vi "Pengukuran WHS 4 Ch.vi"() -> ()   [LabVIEW 2018]
uses:
  <vilib>/Utility/error.llb/DialogType.ctl
  <vilib>/DAQmx/read.llb/DAQmx Read (Analog 1D Wfm NChan NSamp).vi
  <vilib>/DAQmx/configure/timing.llb/DAQmx Timing (Sample Clock).vi
  <vilib>/DAQmx/miscellaneous.llb/DAQmx Fill In Error Info.vi
panel:
  in  "Enable Rekam":bool=TRUE caption="Enable"
  in  "Filename":path=path "D:/Kerjaan Kantor/2019/Studi Banding Lab Pantai Bali - Nov 2019/Uji coba kalibrasi sistem di harbour kolam dalam MOB/validasi.txt"
  in  "Tab Control":enum32{"WHS 4 Channel"}(tab)
  out "Waveform Chart":waveform(dbl)[](graph)
  in  "DAQ Channel":refnum<k21>="WHS_2:5"
  in  "Rate (Hz)":dbl=50.0 format="%0.2f"
  in  "stop":bool
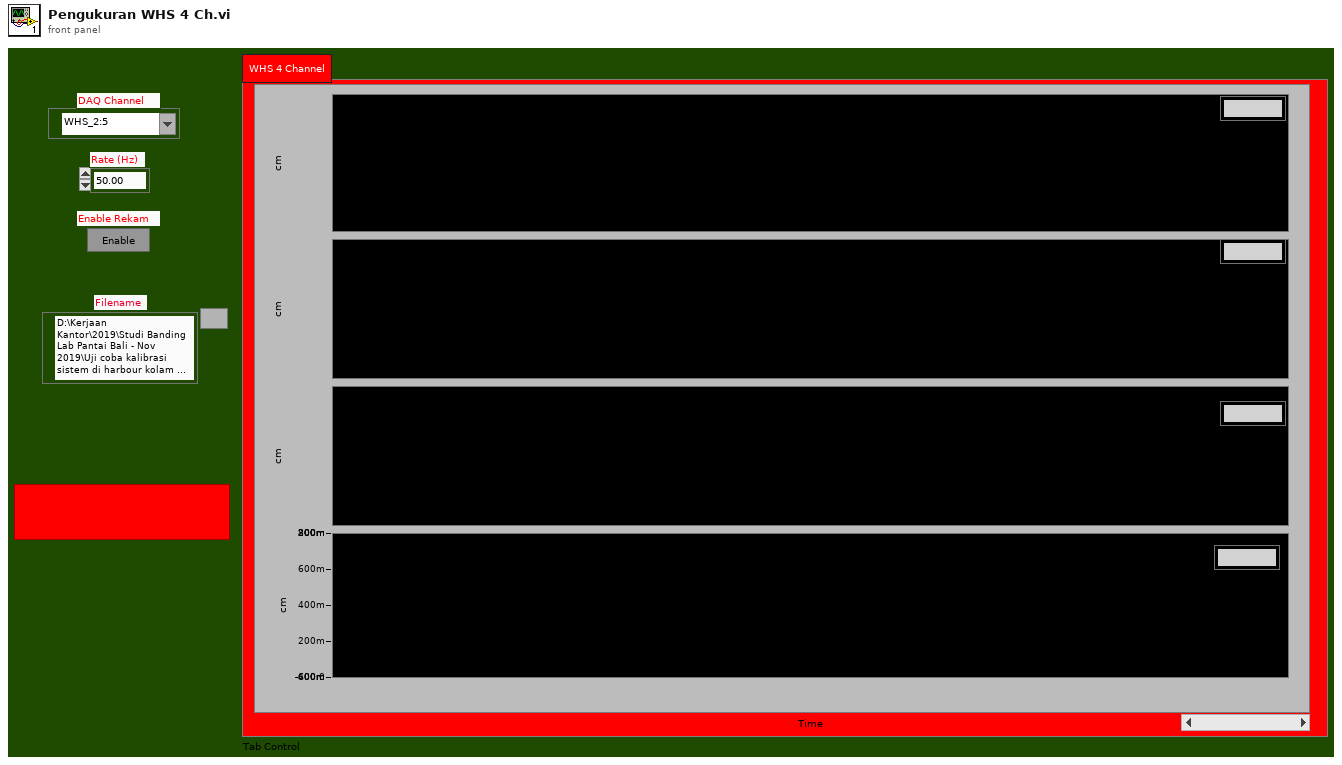
[diagram p1: front panel]
types:
  T1 = typedef "DialogType.ctl" = u16
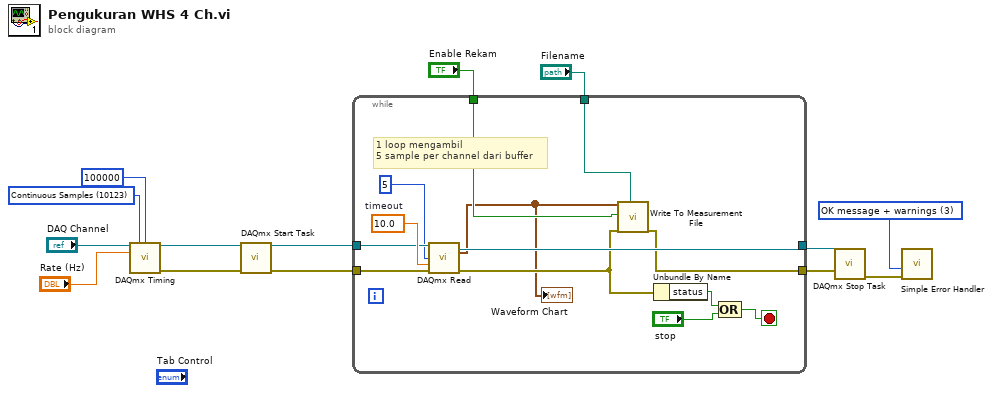
[diagram p0: block diagram]
diagram:
  w13 = 10123 items=["Finite Samples"=10178, "Continuous Samples"=10123, "Hardware Timed Single Point"=12522] ("Sample Mode")
  w10 = T1 3 items=["no dialog", "OK message", "continue or stop message", "OK message + warnings", "continue/stop + warnings"] ("type of dialog (OK msg:1)")
  n1 = call-poly <vilib>:"DAQmx Timing.vi"("task/channels in"="DAQ Channel", "sample mode"=w13, "samples per channel"=100000 ("Max Data/Buffer"), "rate"="Rate (Hz)") -> ("task out"=w12:refnum<k21>, "error out"=w11:errorcluster)  [unwired: 10 in]
  n2 = call <vilib>:"DAQmx Start Task.vi"("task/channels in"=w12, "error in"=w11) -> ("task out"=w2:refnum<k21>, "error out"=w1:errorcluster)  [unwired: 12 in]
  n3 = while {
    tunnel: w1 -> [w26]
    tunnel: w2 -> [w25]
    tunnel: [w20] -> w8
    tunnel: [w22] -> w6
    tunnel: "Filename" -> [w19]
    tunnel: "Enable Rekam" -> [w18]
    stop <- w17 stop-if-true
    w27 = 10.0  # timeout
    # "1 loop mengambil\n5 sample per channel dari buffer"
    n4 = call-poly <vilib>:"DAQmx Read.vi"("task/channels in"=w25, "number of samples per channel"=5, "timeout"=w27, "error in"=w26) -> ("task out"=w22:refnum<k21>, "data"=w16:waveform(dbl)[], "error out"=w21:errorcluster)  [unwired: 9 in]
    "Waveform Chart" <- w16
    n5 = call "Write To Measurement File"("Signals"=w16, "Enable"=w18, "error in (no error)"=w21, "Filename"=w19) -> ("error out"=w20:errorcluster)  [unwired: 13 in, 2 out]
    n6 = Unbundle By Name(w21) -> ("status"=w24:bool)
    n7 = Compound Arithmetic op=OR(w24, "stop") -> (w17:bool)
  }
  n8 = call <vilib>:"DAQmx Stop Task.vi"("task/channels in"=w6, "error in"=w8) -> ("error out"=w9:errorcluster)  [unwired: 12 in, 1 out]
  n9 = call <vilib>:"Simple Error Handler.vi"("type of dialog (OK msg:1)"=w10, "error in (no error)"=w9) -> ()  [unwired: 3 in, 5 out]
